vi "LoadModel.vi"(8 "error in (no error)":errorcluster, 10 "Actor In":refnum<class "Actor.lvclass">, 11 "GRMActor in":refnum<class "StageController.lvclass">) -> (0 "error out":errorcluster, 3 "GRMActor out":refnum<class "StageController.lvclass">)   [LabVIEW 2020, in "StageController.lvlib" / "StageController.lvclass"]
uses:
  StageController.lvclass
  <vilib>/ActorFramework/Actor/Actor.lvclass
  Model/Hardware Layer/Simulation Hardware/DemoStage/DemoStage/DemoStage.lvclass
  D:/Daguan/Development/MMicroscopyFramework/Model/Hardware Abstraction Layer/Component/Stage/Stage/Stage.lvclass
  Model/Hardware Layer/Real Hardware/Stage_MadCityLab/Stage_MadCityLab/Stage_MadCityLab.lvclass
  Model/Hardware Abstraction Layer/Component/Stage/Stage/Stage.lvclass
  C:/Program Files/National Instruments/LabVIEW 2020/vi.lib/ActorFramework/Actor/Actor.lvclass
  Model/Hardware Abstraction Layer/Component/GenericActor/GenericActor/GenericController.lvclass
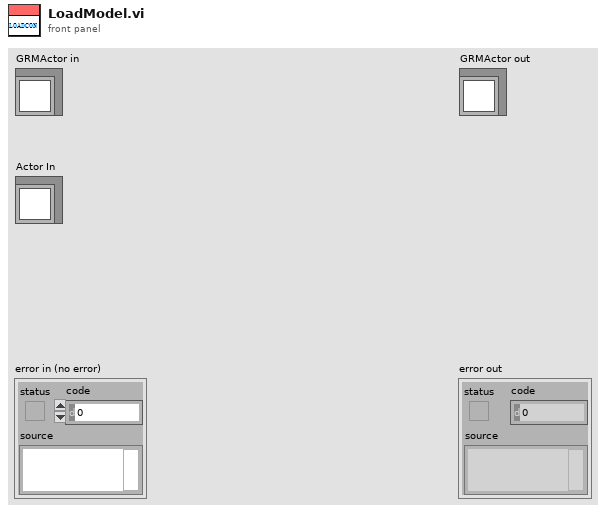
[diagram p1: front panel]
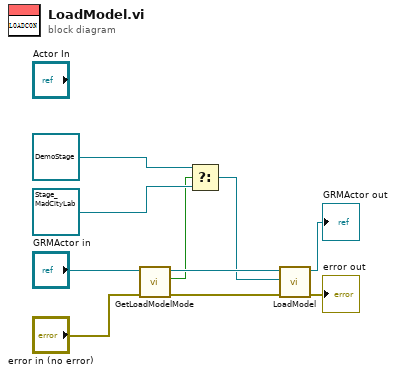
[diagram p0: block diagram]
diagram:
  n1 = call-dynamic "GetLoadModelMode.vi"("error in (no error)"="error in (no error)", "GenericController in"="GRMActor in") -> ("error out"=w7:errorcluster, "LoadDemoModel"=w2:bool, "GenericController out"=w5:refnum<class "StageController.lvclass">)  [unwired: 7 in]
  n2 = Select(t=refnum<class "DemoStage.lvclass"> refnum ("DemoStage.lvlib:DemoStage.lvclass"), s=w2, f=refnum<class "Stage_MadCityLab.lvclass"> refnum ("Stage_MadCityLab.lvlib:Stage_MadCityLab.lvclass")) -> (s? t:f=w1:refnum<class "Stage.lvclass">)
  n3 = call-parent "LoadModel.vi"("error in (no error)"=w7, "Actor In"=w1, "GRMActor in"=w5) -> ("error out"=→"error out":errorcluster, "GRMActor out"=→"GRMActor out":refnum<class "StageController.lvclass">)  [unwired: 7 in]
